vi "Excel_Set_Font_Range.vi"(0 "Excel.Range":refnum<k7>, 2 "font":T1 {"font size" format="%0.2f"; "strike through" items=["Unchanged", "Yes", "No"]; "underline" items=["Unchanged", "Yes", "No"]; "italic" items=["Unchanged", "Yes", "No"]; "bold" items=["Unchanged", "Yes", "No"]}, 3 "error in (no error)":errorcluster) -> (6 "Excel.Range out":refnum<k7>, 9 "error out":errorcluster)   [LabVIEW 2010, in "NI_ReportGenerationToolkit.lvlib"]
uses:
  <vilib>/addons/_office/NI_ReportGenerationToolkit.lvlib
  <vilib>/addons/_office/_exclsub.llb/font.ctl
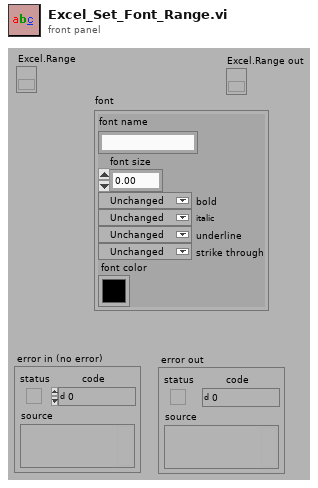
[diagram p1: front panel]
types:
  T1 = typedef "NI_ReportGenerationToolkit.lvlib/font.ctl" = cluster{"font name":string, "font size":dbl, "bold":u16, "italic":u16, "underline":u16, "strike through":u16, "font color":u32}
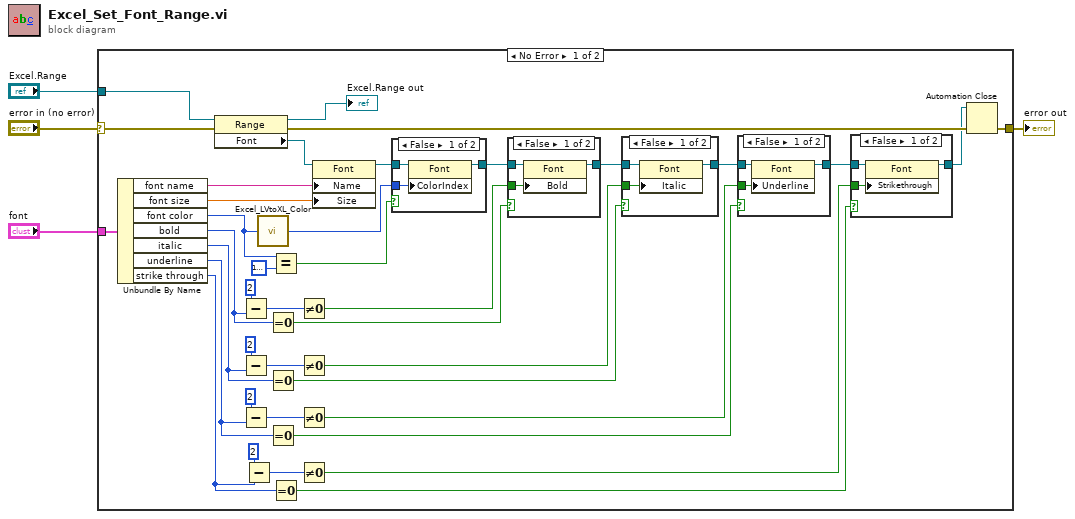
[diagram p0: block diagram]
diagram:
  n1 = case shown="No Error" "error in (no error)" {
    selector: "error in (no error)" -> [w6 w64]
    tunnel: "Excel.Range" -> [w43 _]
    tunnel: [w42 w64] -> w4
    tunnel: "font" -> [w18 _]
    frame No Error {
      n2 = Unbundle By Name(w18) -> ("font name"=w39:string, "font size"=w38:dbl, "font color"=w9:u32, "bold"=w34:u16, "italic"=w24:u16, "underline"=w23:u16, "strike through"=w22:u16)
      n3 = property class="Range"(reference=w43, error in=w6) -> (reference out=→"Excel.Range out":refnum<k7>, error out=w41:errorcluster, "Font"=w40:refnum<k7>)
      n4 = Subtract(x=2, y=w34) -> (x-y=w35:i32)
      n5 = Subtract(x=2, y=w24) -> (x-y=w33:i32)
      n6 = Subtract(x=2, y=w23) -> (x-y=w28:i32)
      n7 = Subtract(x=2, y=w22) -> (x-y=w27:i32)
      n8 = call <vilib>:"Excel_LVtoXL_Color.vi"("LabVIEW color"=w9) -> ("excel color table index"=w8:i32)
      n9 = Equal To 0?(x=w34) -> (x = 0?=w37:bool)
      n10 = Equal To 0?(x=w24) -> (x = 0?=w31:bool)
      n11 = Equal To 0?(x=w23) -> (x = 0?=w30:bool)
      n12 = Equal?(x=w9, y=u32 16777216) -> (x = y?=w10:bool)
      n13 = Equal To 0?(x=w22) -> (x = 0?=w25:bool)
      n14 = Not Equal To 0?(x=w35) -> (x != 0?=w16:bool)
      n15 = Not Equal To 0?(x=w33) -> (x != 0?=w15:bool)
      n16 = Not Equal To 0?(x=w28) -> (x != 0?=w14:bool)
      n17 = Not Equal To 0?(x=w27) -> (x != 0?=w13:bool)
      n18 = property class="Font"(reference=w40, "Name"=w39, "Size"=w38) -> (reference out=w12:refnum<k7>)  [unwired: 1 in, 1 out]
      n19 = case shown="False" w10 {
        tunnel: w12 -> [w46 w47]
        tunnel: w8 -> [w45 _]
        tunnel: [w44 w47] -> w11
        frame False {
          n20 = property class="Font"(reference=w46, "ColorIndex"=w45) -> (reference out=w44:refnum<k7>)  [unwired: 1 in, 1 out]
        }
        frame True {
        }
      }
      n21 = case shown="False" w37 {
        tunnel: w11 -> [w62 w63]
        tunnel: w16 -> [w61 _]
        tunnel: [w60 w63] -> w21
        frame False {
          n22 = property class="Font"(reference=w62, "Bold"=w61) -> (reference out=w60:refnum<k7>)  [unwired: 1 in, 1 out]
        }
        frame True {
        }
      }
      n23 = case shown="False" w31 {
        tunnel: w21 -> [w58 w59]
        tunnel: w15 -> [w57 _]
        tunnel: [w56 w59] -> w20
        frame False {
          n24 = property class="Font"(reference=w58, "Italic"=w57) -> (reference out=w56:refnum<k7>)  [unwired: 1 in, 1 out]
        }
        frame True {
        }
      }
      n25 = case shown="False" w30 {
        tunnel: w20 -> [w54 w55]
        tunnel: w14 -> [w53 _]
        tunnel: [w52 w55] -> w19
        frame False {
          n26 = property class="Font"(reference=w54, "Underline"=w53) -> (reference out=w52:refnum<k7>)  [unwired: 1 in, 1 out]
        }
        frame True {
        }
      }
      n27 = case shown="False" w25 {
        tunnel: w19 -> [w50 w51]
        tunnel: w13 -> [w49 _]
        tunnel: [w48 w51] -> w17
        frame False {
          n28 = property class="Font"(reference=w50, "Strikethrough"=w49) -> (reference out=w48:refnum<k7>)  [unwired: 1 in, 1 out]
        }
        frame True {
        }
      }
      n29 = Automation Close(3:w41, 5:w17) -> (0:w42:errorcluster)
    }
    frame Error {
    }
  }
  "error out" <- w4
